vi "Create Frame Pattern Script.vi"(8 "error in (no error)":errorcluster, 9 "ChipID":u8, 10 "Frame_Data":T1={"Pattern_Name"="", "Operation Mode"=enum."Normal", "BurstLength"=enum."0", "FSN"=0, "Start_Addr"=0, "Data"=[], "R/W?"=enum."Read", "Opcode"=[], "ChipID"=1, "num of wait cycle of read"=0} {"Data" format="%x"; "Start_Addr" format="%x"}, 11 "BML_Frame_Read in":refnum<class "BML_Frame_Read.lvclass">) -> (0 "error out":errorcluster, 3 "BML_Frame_Read out":refnum<class "BML_Frame_Read.lvclass">)   [LabVIEW 2018, in "BML_Frame_Read.lvclass"]
uses:
  BML_Frame_Read.lvclass
  C:/P4 Workspace/PC Client/Solutions/5g_eap/HiSi/trunk/1.0/BML_Pattern_Gen_Refactor/Classes/BML_Frame_Root/BML_Frame_Root.lvclass
  Config_Read/Frame_Data.ctl
  Config_Read/OperationMode.ctl
  Config_Read/BurstLength.ctl
  Config_Read/RW_Option.ctl
  BML_Frame_Read.lvclass/BML_Frame_Read.ctl
  BML_Frame_Root/BML_Frame_Root.lvclass/BML_Frame_Root.ctl
  BML_Frame_ReadCollect/BML_Frame_ReadCollect.lvclass
  BML_Frame_ReadData_Value_Cap/BML_Frame_ReadData_ValueCap.lvclass
  Config_Read/Config_Read_BML.lvclass
  BML_Frame_Root/BML_Frame_Root.lvclass
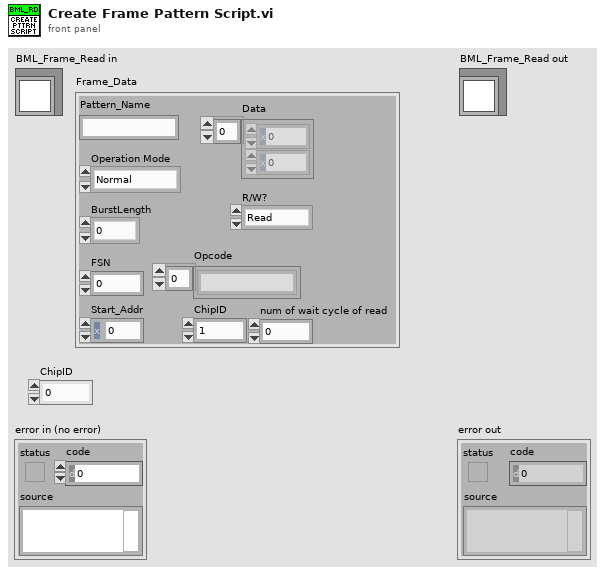
[diagram p1: front panel]
types:
  T1 = typedef "Config_Read_BML.lvclass/Frame_Data.ctl" = cluster{"Pattern_Name":string, "Operation Mode":T2, "BurstLength":T3, "FSN":u8, "Start_Addr":u16, "Data":u8[], "R/W?":T4, "Opcode":string[], "ChipID":u8, "num of wait cycle of read":i8}
  T2 = typedef "Config_Read_BML.lvclass/OperationMode.ctl" = enum8{"Normal", "ImmeEffect", "InitSlaveID", "LoadData"}
  T3 = typedef "Config_Read_BML.lvclass/BurstLength.ctl" = enum8{"0", "2", "3", "4", "5", "8", "16", "32"}
  T4 = typedef "Config_Read_BML.lvclass/RW_Option.ctl" = enum16{"Read", "Write", "R/W"}
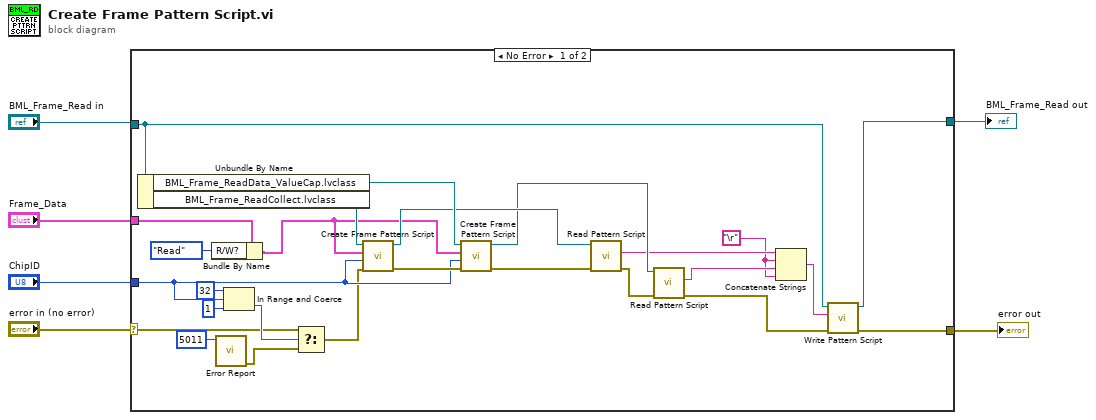
[diagram p0: block diagram]
diagram:
  n1 = case shown="No Error" "error in (no error)" {
    selector: "error in (no error)" -> [w13 w34]
    tunnel: [w21 w34] -> w1
    tunnel: "BML_Frame_Read in" -> [w23 w33]
    tunnel: [w22 w33] -> w2
    tunnel: "Frame_Data" -> [w20 _]
    tunnel: "ChipID" -> [w14 _]
    frame No Error {
      w24 = "\r"
      n2 = Unbundle By Name(w23) -> ("BML_Frame_ReadData_ValueCap.lvclass"=w30:refnum<class "BML_Frame_ReadData_ValueCap.lvclass">, "BML_Frame_ReadCollect.lvclass"=w31:refnum<class "BML_Frame_ReadCollect.lvclass">)
      n3 = Bundle By Name(cluster=w20, "R/W?"=RW_Option."Read") -> (w18:T1)
      n4 = call "Error Report.vi"("Error Code"=i16 5011) -> ("error out"=w12:errorcluster)  [unwired: 10 in]
      n5 = In Range and Coerce(upper limit=u8 32, x=w14, lower limit=u8 1) -> (In Range?=w16:bool)  [unwired: 1 out]
      n6 = Select(t=w13, s=w16, f=w12) -> (s? t:f=w11:errorcluster)
      n7 = call-dynamic "Create Frame Pattern Script.vi"("error in (no error)"=w11, "ChipID"=w14, "Frame_Data"=w18, "BML_Frame_ReadCollect in"=w31) -> ("error out"=w32:errorcluster, "BML_Frame_ReadCollect out"=w29:refnum<class "BML_Frame_ReadCollect.lvclass">)  [unwired: 6 in]
      n8 = call-dynamic "Create Frame Pattern Script.vi"("error in (no error)"=w32, "ChipID"=w14, "Frame_Data"=w18, "BML_Frame_ReadData_ValueCap in"=w30) -> ("error out"=w9:errorcluster, "BML_Frame_ReadData_ValueCap out"=w27:refnum<class "BML_Frame_ReadData_ValueCap.lvclass">)  [unwired: 6 in]
      n9 = call "Read Pattern Script.vi"("error in (no error)"=w9, "BML_Frame_Root in"=w29) -> ("error out"=w28:errorcluster, "Pattern Script"=w26:string)  [unwired: 7 in, 1 out]
      n10 = call "Read Pattern Script.vi"("error in (no error)"=w28, "BML_Frame_Root in"=w27) -> ("error out"=w8:errorcluster, "Pattern Script"=w25:string)  [unwired: 7 in, 1 out]
      n11 = Concatenate Strings(w26, w24, w25, w24) -> (w7:string)
      n12 = call "Write Pattern Script.vi"("error in (no error)"=w8, "Pattern Script"=w7, "BML_Frame_Root in"=w23) -> ("error out"=w21:errorcluster, "BML_Frame_Root out"=w22:refnum<class "BML_Frame_Read.lvclass">)  [unwired: 7 in]
    }
    frame Error {
    }
  }
  "error out" <- w1
  "BML_Frame_Read out" <- w2
